vi "Get Available MetaData Channels.vi"(8 "error in (no error)":errorcluster, 10 "MetaData":refnum<vi>, 11 "Item Ref in":T1 format="%.0x") -> (0 "error out":errorcluster, 3 "Item Ref out":T1 format="%.0x")   [LabVIEW 2019, in "Instrument Addon System Explorer.lvlib"]
uses:
  Instrument Addon System Explorer.lvlib
  <vilib>/NI VeriStand/Custom Device API/Custom Device API.lvlib
  <vilib>/NI VeriStand/Custom Device API/Get Item Property (String).vi
  Addon Shared/SubVIs/Constants.vi
  Addon Shared/Instrument Addon Shared.lvlib
  <vilib>/Utility/miscctls.llb/LVComboBoxStrsAndValuesArrayTypeDef.ctl
  <vilib>/NI VeriStand/Custom Device API/Custom Device Item Ref.ctl
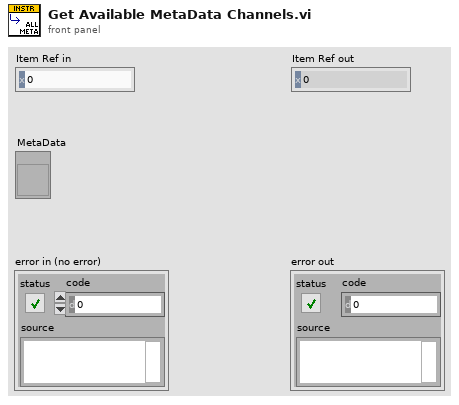
[diagram p1: front panel]
types:
  T1 = typedef "Custom Device API.lvlib/Custom Device Item Ref.ctl" = u64
  T2 = typedef "LVComboBoxStrsAndValuesArrayTypeDef.ctl" = cluster{"String":string, "Value":string}[]
  T3 = typedef "Custom Device API.lvlib/Custom Device Item Info.ctl" = cluster{"Name":string, "Is Channel":bool, "GUID":string, "Is Waveform":bool}
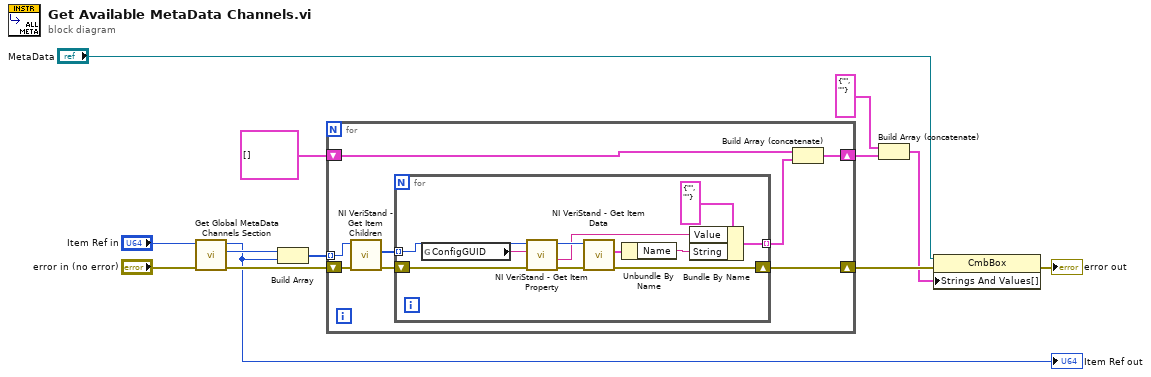
[diagram p0: block diagram]
diagram:
  n1 = call "Get Global MetaData Channels Section.vi"("error in (no error)"="error in (no error)", "Item Ref in"="Item Ref in") -> ("error out"=w9:errorcluster, "Item Ref"=w3:T1, "Item Ref out"=w1:T1)  [unwired: 7 in]
  "Item Ref out" <- w1
  n2 = Build Array(w3, w1) -> (w8:T1[])
  n3 = for {
    tunnel: w8 -> [w16] mode=indexing
    shift-right: [w15] -> w13
    shift-left: T2 [] ("Strings And Values []") -> [w14]
    shift-right: [w20] -> w11
    shift-left: w9 -> [w17]
    n4 = call <vilib>:"NI VeriStand - Get Item Children.vi"("error in (no error)"=w17, "Item Ref in"=w16) -> ("error out"=w18:errorcluster, "Child Refs"=w19:T1[])  [unwired: 6 in, 2 out]
    n5 = for {
      tunnel: w19 -> [w31] mode=indexing
      shift-right: [w30] -> w20
      shift-left: w18 -> [w27]
      tunnel: [w29] -> w21 mode=indexing
      n6 = global read "Constants.vi" "ConfigGUID"() -> (w25:string)
      n7 = call-poly <vilib>:"NI VeriStand - Get Item Property.vi"("error in (no error)"=w27, "Property Name"=w25, "Item Ref in"=w31) -> ("error out"=w26:errorcluster, "Value"=w23:string, "Item Ref out"=w28:T1)  [unwired: 5 in, 1 out]
      n8 = call <vilib>:"NI VeriStand - Get Item Data.vi"("error in (no error)"=w26, "Item Ref in"=w28) -> ("error out"=w30:errorcluster, "Item Info"=w32:T3)  [unwired: 8 out]
      n9 = Unbundle By Name(w32) -> ("Name"=w22:string)
      n10 = Bundle By Name(cluster=cluster{"String":string, "Value":string} {"String"="", "Value"=""}, "Value"=w23, "String"=w22) -> (w29:cluster{"String":string, "Value":string})
    }
    n11 = Build Array (concatenate)(w14, w21) -> (w15:T2)
  }
  n12 = Build Array (concatenate)(cluster{"String":string, "Value":string} {"String"="", "Value"=""}, w13) -> (w4:T2)
  n13 = property class="CmbBox"(reference="MetaData", error in=w11, "Strings And Values[]"=w4) -> (error out=→"error out":errorcluster)  [unwired: 1 out]
